vi "ROS_Topic_Close_Primitive.vi"(2 "error in":errorcluster, 3 "ROS in":T1) -> (0 "error out":errorcluster)   [LabVIEW 2013]
uses:
  SubVIs/_ROSControl.ctl
  SubVIs/_ROSDirection.ctl
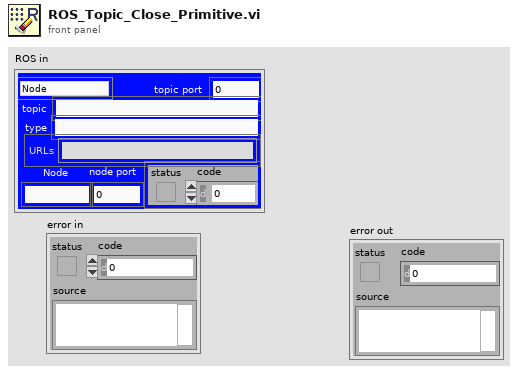
[diagram p1: front panel]
types:
  T1 = typedef "_ROSControl.ctl" = cluster{"topic port":u16, "Node":string, "topic":string, "type":string, "node port":u32, "error ":errorcluster, "Direction":T2, "APIs":string[]}
  T2 = typedef "_ROSDirection.ctl" = enum16{"Node", "Publisher", "Subscriber", "Service Client"}
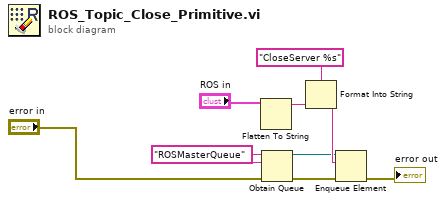
[diagram p0: block diagram]
diagram:
  w8 = "ROSMasterQueue" ("name (unnamed)")
  n1 = Flatten To String(anything="ROS in") -> (data string=w4:string)  [unwired: 3 in, 2 out]
  n2 = Obtain Queue(name (unnamed)=w8, element data type=w8, error in (no error)="error in") -> (queue out=w5:refnum<queue>, error out=w3:errorcluster)  [unwired: 2 in, 1 out]
  n3 = Format Into String(format string="CloseServer %s", w4) -> (resulting string=w6:string)  [unwired: 2 in, 1 out]
  n4 = Enqueue Element(queue=w5, element=w6, error in (no error)=w3) -> (error out=→"error out":errorcluster)  [unwired: 1 in, 2 out]
